vi "Dashboard Main.vi"() -> ()   [LabVIEW 2017]
uses:
  <vilib>/Utility/miscctls.llb/LVRowAndColumnTypeDef.ctl
  <vilib>/event_ctls.llb/eventvkey.ctl
  <vilib>/Rock Robotics/Network Tables/NT Read Numeric Array.vi
  <vilib>/Rock Robotics/WPI/Dashboard/WPI_DashboardLogging Global.vi
panel:
  in  "Camera Settings Right":T1={"Frame Rate"=30, "Compression"=30, "Size"=1, "DB Camera Config"=FALSE} {"Frame Rate" scale=1.0..30.0; "Compression" scale=100.0..-1.0; "Size" items=["640x480", "320x240", "160x120"]}
  in  "Camera Name Right":string(combo)="No Camera Selection"
  out "Camera Info":cluster{"Mbps LED":bool, "Mbps":dbl, "fps":dbl} {"fps" format="%#.1g"; "Mbps" format="%#.1g"}
  in  "Camera Settings":T1={"Frame Rate"=30, "Compression"=30, "Size"=1, "DB Camera Config"=FALSE} {"Frame Rate" scale=1.0..30.0; "Compression" scale=100.0..-1.0; "Size" items=["640x480", "320x240", "160x120"]}
  in  "TCP":refnum<k5>
  in  "Rec Mode":enum32{"Stop", "Record", "Playback"}(radio)
  out "Robot IP":string
  out "Image Message":string="Timeout in Camera Communications"
  in  "Dashboard Tab":T2(tab)
  in  "Select Auto":string(combo)="Select Autonomous ..."
  out "NT Connection":bool
  out "MotorChart R":cluster{"Numeric":dbl, "Numeric":dbl}(graph)
  out "MotorChart L":cluster{"Numeric":dbl, "Numeric":dbl}(graph)
  out "MotorSliders R":cluster{"MotorSlide1":dbl, "MotorSlide2":dbl} {"MotorSlide2" scale=-1.0..1.0 scale format="%#_2e"; "MotorSlide1" scale=-1.0..1.0 scale format="%#_2e"}
  out "MotorSliders L":cluster{"MotorSlide1":dbl, "MotorSlide2":dbl} {"MotorSlide2" scale=-1.0..1.0 scale format="%#_2e"; "MotorSlide1" scale=-1.0..1.0 scale format="%#_2e"}
  out "JS1 Z":dbl(slide) scale=-1.0..1.0 scale format="%#_2e"
  out "JS1 Graph":cluster{"X":dbl, "Y":dbl}[](graph)
  out "JS1 Buttons":T3
  out "JS2 Z":dbl(slide) scale=-1.0..1.0 scale format="%#_2e"
  out "JS2 Graph":cluster{"X":dbl, "Y":dbl}[](graph)
  out "JS2 Buttons":T3
  out "Mode":T4(ring)=enum."Auto Disabled"
  out "Gear State":string="Waiting...."
  out "Camera Image Right":T5(plugin-control)
  in  "DB/String 9":string
  in  "DB/String 8":string
  in  "DB/String 7":string
  in  "DB/String 6":string
  in  "DB/String 5":string
  in  "DB/String 4":string
  in  "DB/String 3":string
  in  "DB/String 2":string
  in  "DB/String 1":string
  in  "DB/String 0":string
  in  "DB/Slider 0":dbl(slide) scale=0.0..5.0
  in  "DB/Slider 1":dbl(slide) scale=0.0..5.0
  in  "DB/Slider 2":dbl(slide) scale=0.0..5.0
  in  "DB/Slider 3":dbl(slide) scale=0.0..5.0
  out "DB/LED 3":bool
  out "DB/LED 2":bool
  out "DB/LED 1":bool
  out "DB/LED 0":bool
  in  "DB/Button 3":bool
  in  "DB/Button 2":bool
  in  "DB/Button 1":bool
  in  "DB/Button 0":bool caption="New Name"
  in  "Test Slider":dbl(slide) scale=0.0..100.0 scale format="%#_3g"
  in  "On/Off":bool caption="Solenoid"
  in  "Test Name":u16(ring) items=["Select the test to run..."]
  in  "Test Tree":string(tree)
  in  "Motor":cluster{"Value":dbl, "Enable":bool} {"Value" scale=-1.0..1.0 scale format="%#_3g"}
  out "Progress":T6 {"Test Progress" scale=0.0..100.0}
  in  "Rev/Fwd":cluster{"Forward":bool, "Reverse":bool}
  in  "Test Ring":u16(ring) items=["Monochrome", "Color"]
  out "Cmd Status":string
  in  "Execute Command":bool
  in  "Command Params":string[][](table)
  in  "Command Selection":i32(listbox)
  in  "CheckList":i32(listbox)
  out "Tree":string(tree)
  out "Camera Image":T5(plugin-control)
  out "Background":bool
  in  "Camera Name":string(combo)="No Camera Selection"
  # "HW"
  # "HW"
  # "Joysticks"
  # "Drive Motors"
  # "Front"
  # "Right"
  # "Left"
  # "Back"
  # "This tab is a great place for autonomous settings and robot-specific values.\nPlace controls and indicators inside this tab and match name to\nDashboard Variables on robot. You can also delete this comment."
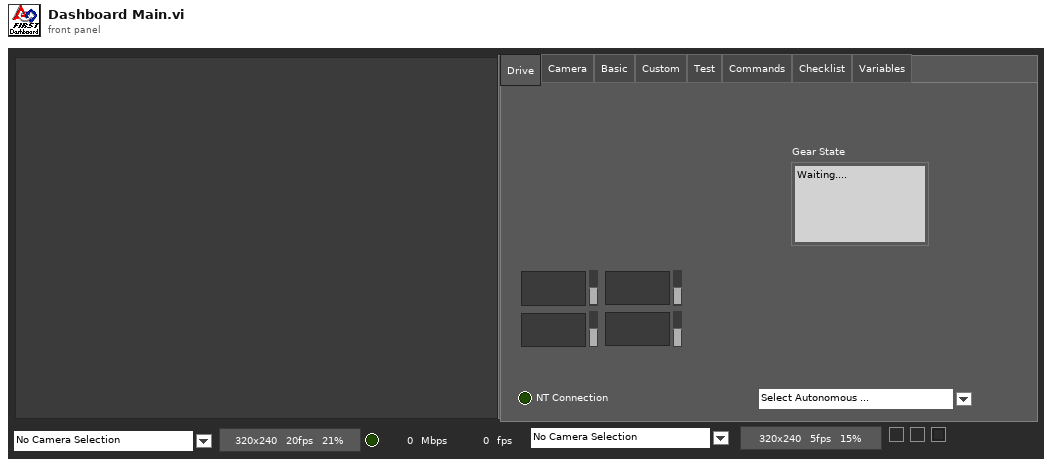
[diagram p1: front panel]
types:
  T1 = cluster{"Frame Rate":i32, "Compression":i32, "Size":u16, "DB Camera Config":bool}
  T2 = enum32{"Drive", "Camera", "Basic", "Custom", "Test", "Commands", "Checklist", "Variables"}
  T3 = cluster{bool, bool, bool, bool, bool, bool, bool, bool, bool, bool, bool, bool}
  T4 = enum8{"Tele-Op Disabled", "Tele-Op Enabled", "Auto Disabled", "Auto Enabled", "Test Disabled", "Test Enabled", "Disconnected", "No Code", "E-Stop"}
  T5 = typedef "IMAQ Image.ctl" = refnum<image>
  T6 = cluster{"Test Progress":u8, "Test Progress Text":string}
  T7 = cluster{"Save Path":path, "Interval (s)":dbl, "Keep":i32}
  T8 = typedef "Image Type" = u32
  T9 = cluster{"IDs":cluster{"RPC field ID":u16, "Unique ID":u16}, "String":string}
  T10 = cluster{"Error Strings":string, "Disable Counts":cluster{u16, u16}, "Rail Faults":cluster{u16, u16, u16}, "Robot IP":string, "DB Mode":u8, "Event Info":cluster{"Name":string, "Type":u8, "Number":u16, "Replay":u8}}
  T11 = cluster{"Storage":cluster{"Disk Free":u64, "RAM Block":u32, "RAM free":u32}, "CPU Utilization":cluster{"CPU % ISR":sgl, "CPU % Time Crit":sgl, "CPU % Timed Str":sgl, "CPU % High":sgl, "CPU % Above":sgl, "CPU % Normal":sgl, "CPU % Low":sgl}, "CAN":cluster{"% Bus Utilization":sgl, "Bus Off Cnt":u32, "TX_FIFO Full Cnt":u32, "Receive Error Cnt":u8, "Transmit Error Cnt":u8}, "HID":cluster{"HID Outputs":u32, "Rumble Low":u16, "Rumble High":u16}[]}
  T12 = cluster{"Status bits":cluster{"Test Mode":bool, "Autonomous":bool, "Enabled":bool, "Code Start":bool, "Brownout":bool, "Reserved 2":bool, "Reserved 3":bool, "E-Stop":bool}, "Code Trace":cluster{"Disabled":bool, "TeleOp":bool, "Auto":bool, "Test":bool}, "Controller Type":enum16{"unknown", "cRIO", "roboRio"}, "Code?":enum16{"unknown", "noCode", "code"}, "Battery V":dbl}
  T13 = cluster{"Control Bits":cluster{"TestMode":bool, "Autonomous":bool, "Enabled":bool, "FMS Present":bool, bool, bool, bool, "E-Stop":bool}, "Team Station ":u8, "Countdown":sgl, "Joystick Values":cluster{"Axes":dbl[], "Buttons":bool[], "POVs":i16[]}[]}
  T14 = cluster{"Axes":dbl[], "Buttons":bool[], "POVs":i16[]}[]
  T15 = cluster{"Axes":dbl[], "Buttons":bool[], "POVs":i16[]}
  T16 = cluster{"Buttons[0]":bool, "Buttons[1]":bool, "Buttons[2]":bool, "Buttons[3]":bool, "Buttons[4]":bool, "Buttons[5]":bool, "Buttons[6]":bool, "Buttons[7]":bool, "Buttons[8]":bool, "Buttons[9]":bool, "Buttons[10]":bool, "Buttons[11]":bool}
  T17 = cluster{"Camera Image":refnum<vi>, "Dashboard Tab":refnum<vi>, "Background":refnum<vi>, "Rec Mode":refnum<vi>, "Test Slider":refnum<vi>, "On/Off ":refnum<vi>, "Test Ring":refnum<vi>, "Rev/Fwd":refnum<vi>, "Test Name":refnum<vi>, "Motor":refnum<vi>, "Progress":refnum<vi>, "CheckList":refnum<vi>, "Tree":refnum<vi>, "Test Tree":refnum<vi>, "Command Params":refnum<vi>, "Command Selection":refnum<vi>, "Execute Command":refnum<vi>, "Cmd Status":refnum<vi>, "Camera Settings":refnum<vi>, "Camera Name":refnum<vi>, "Camera Info":refnum<vi>, "Camera Settings Right":refnum<vi>, "Camera Name Right":refnum<vi>, "Camera Image Right":refnum<vi>}
  T18 = cluster{"Camera Name":string, string, "Saved DB Images Info":cluster{"Save Path":path, "Interval (s)":dbl, "Keep":i32}}
  T19 = cluster{"Camera Name Right":string, string, "Saved DB Images Info":cluster{"Save Path":path, "Interval (s)":dbl, "Keep":i32}}
  T20 = cluster{"Operation":enum16{"Update", "Clear"}, "Color Box":u32}[]
  T21 = typedef "eventvkey.ctl" = enum16{"ASCII", "Enter", "Return", "Shift", "Ctrl", "Alt", "Cmd", "Opt", "Caps", "NumLock", "Clear", "Break", "Up", "Down", "Left", "Right", "Insert", "Delete", "Home", "End", "PageUp", "PageDown", "Escape", "Help", "Pause", "ScrollLock", "F1", "F2", "F3", "F4", "F5", "F6", "F7", "F8", "F9", "F10", "F11", "F12", "F13", "F14", "F15", "F16", "F17", "F18", "F19", "F20", "F21", "F22", "F23", "F24", "Play", "VolumeUp", "VolumeDown", "Mute", "Two Byte Char"}
  T22 = cluster{"Image Size":bool, "Image Type":bool, "Pixel Value":bool, "ROI Information":bool, "Zoom Factor":bool}
  T23 = cluster{"Operation":enum16{"Update", "Clear"}, "Color Box":u32}
  T24 = typedef "LVRowAndColumnTypeDef.ctl" = cluster{"Row":i32, "Column":i32}
  T25 = cluster{"Shift":bool, "Ctrl":bool, "Alt":bool, "Cmd":bool, "Opt":bool}
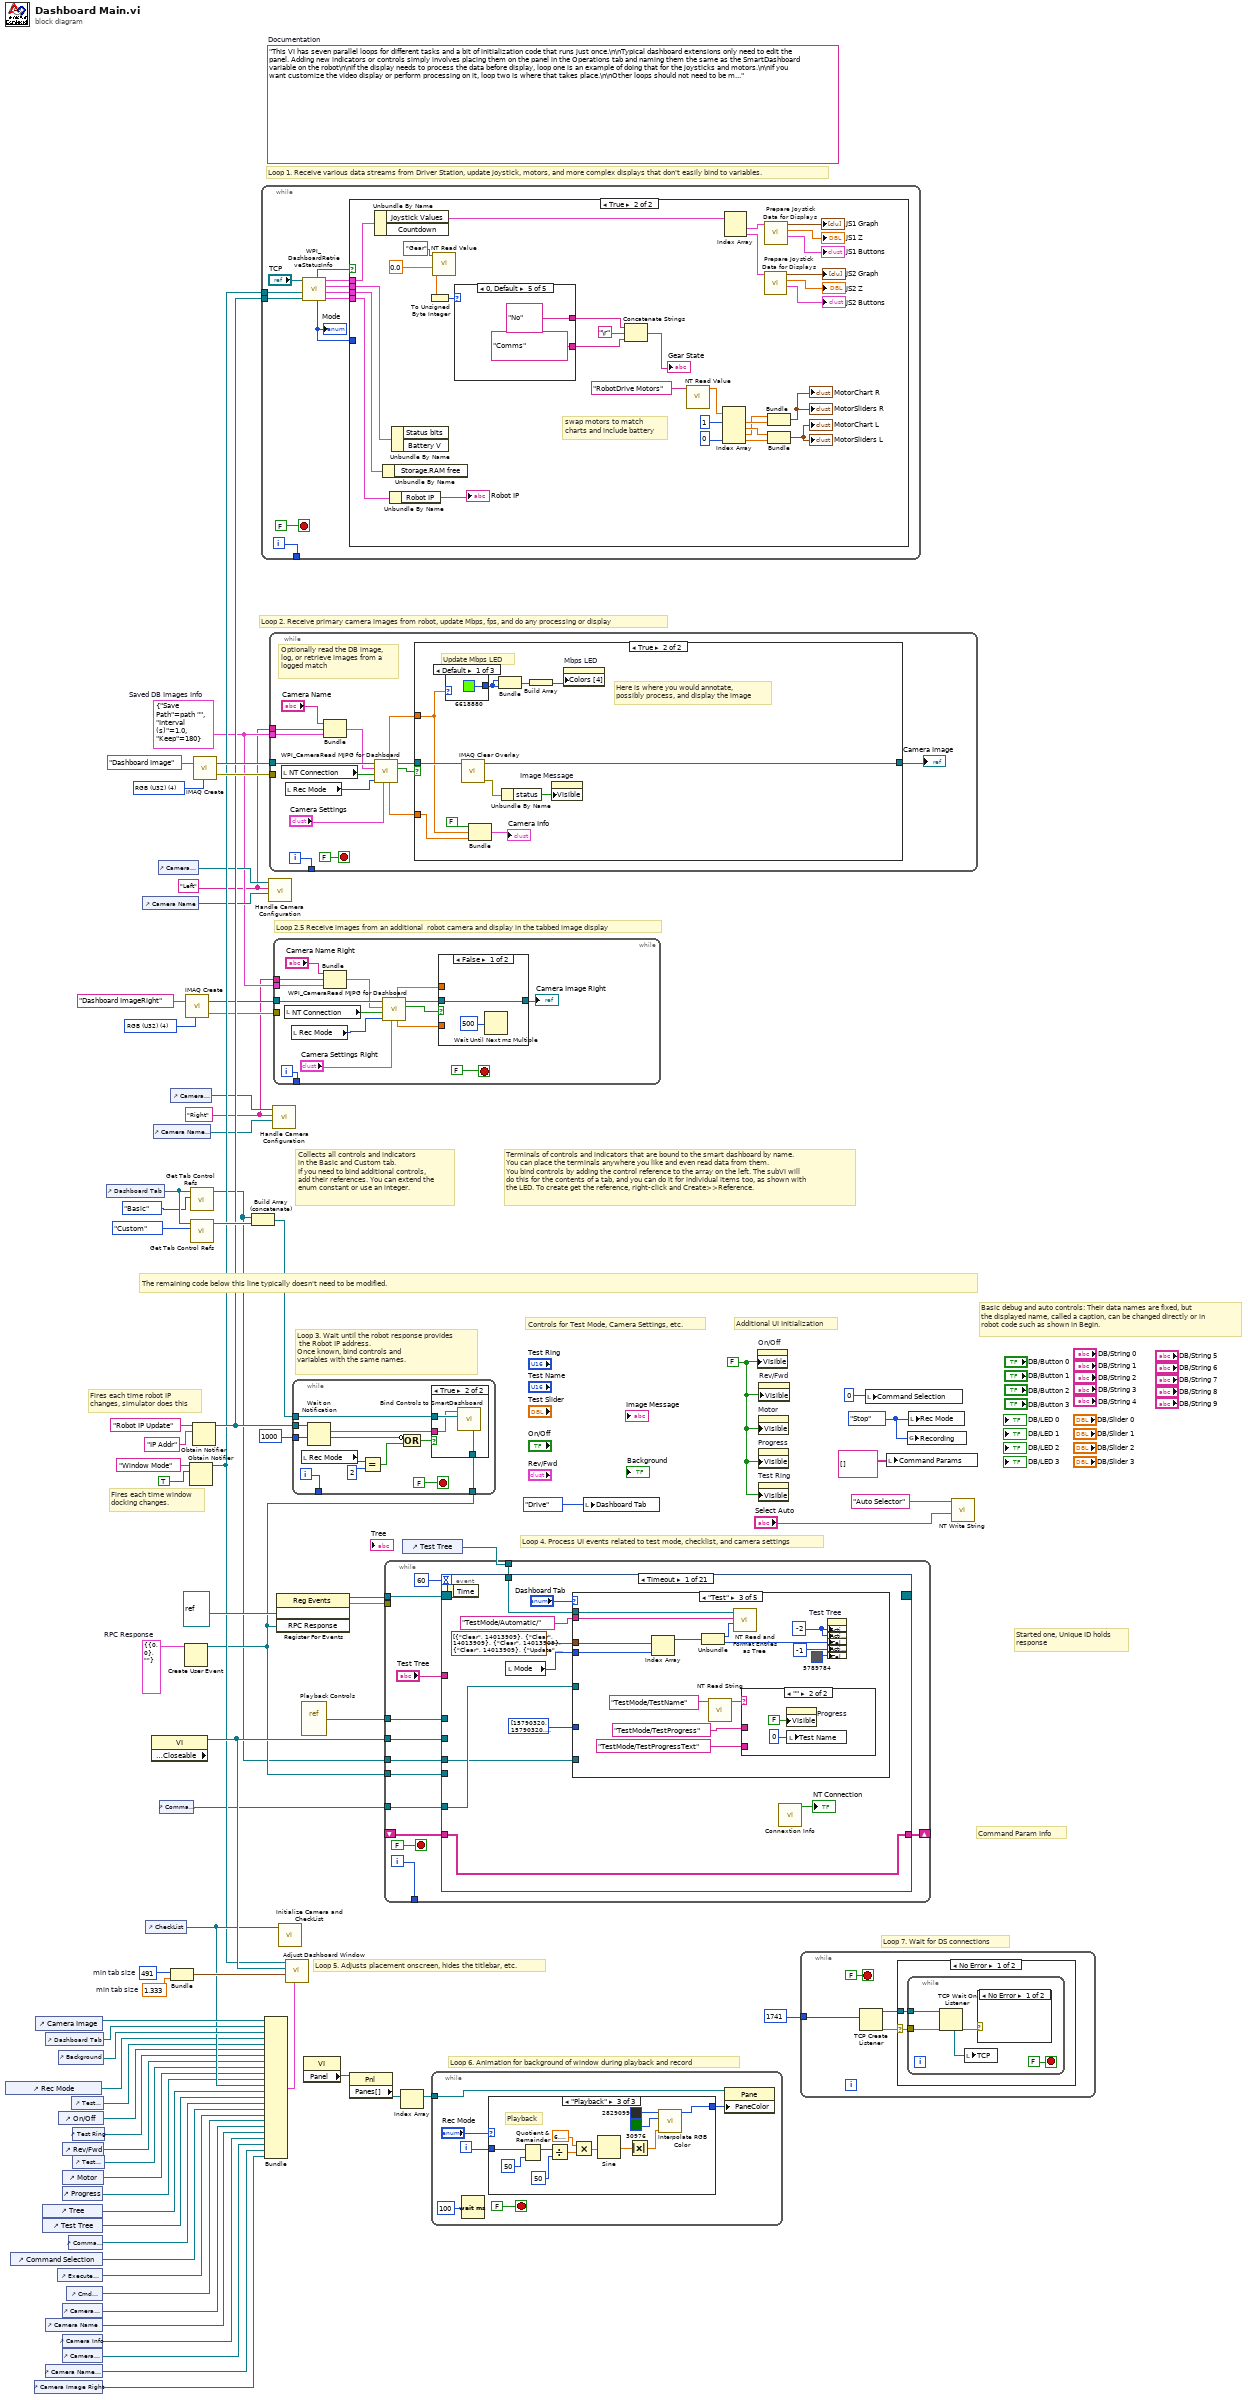
[diagram p0: block diagram]
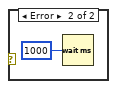
[diagram p3: hidden frame]
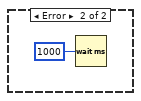
[diagram p4: hidden frame]
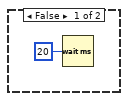
[diagram p5: hidden frame]
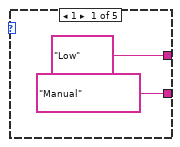
[diagram p6: hidden frame]
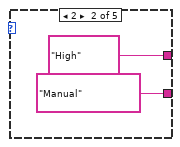
[diagram p7: hidden frame]
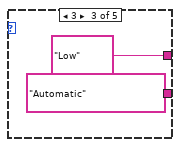
[diagram p8: hidden frame]
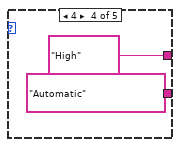
[diagram p9: hidden frame]
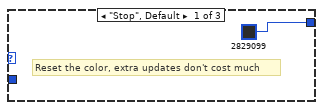
[diagram p10: hidden frame]
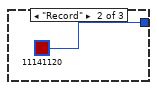
[diagram p11: hidden frame]
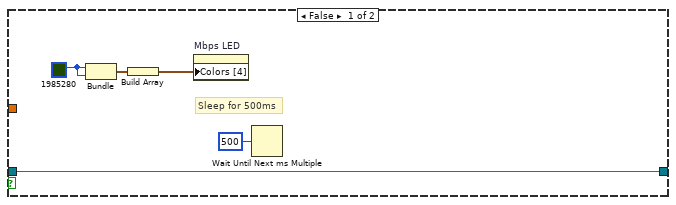
[diagram p13: hidden frame]
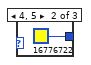
[diagram p14: hidden frame]
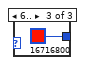
[diagram p15: hidden frame]
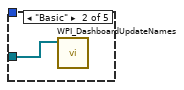
[diagram p17: hidden frame]
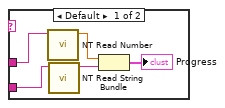
[diagram p18: hidden frame]
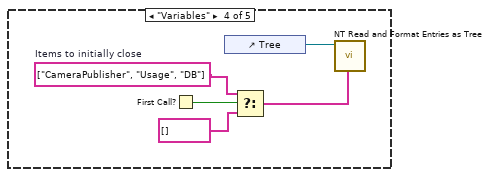
[diagram p19: hidden frame]
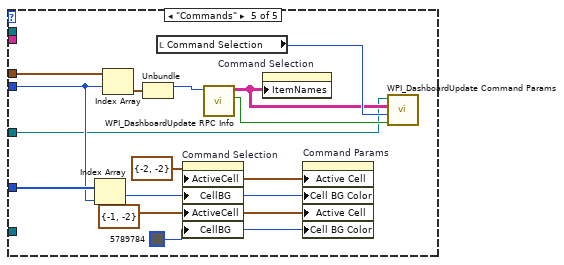
[diagram p20: hidden frame]
diagram:
  w3 = T7 {"Save Path"=path "", "Interval (s)"=1.0, "Keep"=180}  # Saved DB Images Info
  w2 = "Right"
  w1 = "Left"
  w13 = T8 4 items=["Grayscale (U8)", "Grayscale (I16)", "Grayscale (SGL)", "Complex (CSG)", "RGB (U32)", "HSL (U32)", "RGB (U64)"] ("Image Type")
  w29 = T9 {"IDs"={"RPC field ID"=0, "Unique ID"=0}, "String"=""}  # RPC Response
  w52 = 491  # min tab size
  w51 = 1.333  # min tab size
  w59 = enum32{"Stop", "Record", "Playback"}."Stop" ("Rec Mode")
  w36 = FALSE ("Visible")
  (unwired) "This VI has seven parallel loops for different tasks and a bit of initialization code that runs just once.\n\nTypical dashboard extensions only need to edit the panel. Adding new indicators or controls simply involves placing them on the panel in the Operations tab and naming them the same as the SmartDashboard variable on the robot\n\nIf the display needs to process the data before display, loop one is an example of doing that for the joysticks and motors.\n\nIf you want customize the video display or perform processing on it, loop two is where that takes place.\n\nOther loops should not need to be modified. They are pretty standard, and document the task they perform."  # Documentation
  w76 = T8 4 items=["Grayscale (U8)", "Grayscale (I16)", "Grayscale (SGL)", "Complex (CSG)", "RGB (U32)", "HSL (U32)", "RGB (U64)"] ("Image Type")
  # "Loop 2.5 Receive images from an additional  robot camera and display in the tabbed image display"
  # "Command Param Info"
  # "Started one, Unique ID holds\nresponse"
  # "Loop 7. Wait for DS connections"
  # "Basic debug and auto controls: Their data names are fixed, but\nthe displayed name, called a caption, can be changed directly or in\nrobot code such as shown in Begin."
  # "Controls for Test Mode, Camera Settings, etc."
  # "Additional UI Initialization"
  # "Loop 6. Animation for background of window during playback and record"
  # "Fires each time robot IP\nchanges, simulator does this"
  # "Fires each time window\ndocking changes."
  # "Collects all controls and indicators\nin the Basic and Custom tab.\nIf you need to bind additional controls,\nadd their references. You can extend the\nenum constant or use an integer."
  # "The remaining code below this line typically doesn't need to be modified."
  # "Loop 4. Process UI events related to test mode, checklist, and camera settings"
  # "Terminals of controls and indicators that are bound to the smart dashboard by name.\nYou can place the terminals anywhere you like and even read data from them.\nYou bind controls by adding the control reference to the array on the left. The subVI will\ndo this for the contents of a tab, and you can do it for individual items too, as shown with\nthe LED. To create get the reference, right-click and Create>>Reference."
  # "Loop 3. Wait until the robot response provides\n the Robot IP address.\nOnce known, bind controls and\nvariables with the same names."
  # "Loop 5. Adjusts placement onscreen, hides the titlebar, etc."
  # "Loop 1. Receive various data streams from Driver Station, update joystick, motors, and more complex displays that don't easily bind to variables."
  # "Loop 2. Receive primary camera images from robot, update Mbps, fps, and do any processing or display"
  n1 = control-ref of="Rec Mode"() -> (w42:refnum<vi>)
  n2 = control-ref of="Command Selection"() -> (w28:refnum<vi>)
  n3 = control-ref of="Camera Image Right"() -> (w6:refnum<vi>)
  n4 = control-ref of="Camera Image"() -> (w54:refnum<vi>)
  n5 = control-ref of="Tree"() -> (w46:refnum<vi>)
  n6 = control-ref of="Test Tree"() -> (w45:refnum<vi>)
  n7 = control-ref of="Dashboard Tab"() -> (w53:refnum<vi>)
  n8 = control-ref of="Camera Name"() -> (w19:refnum<vi>)
  n9 = control-ref of="Camera Name Right"() -> (w7:refnum<vi>)
  n10 = control-ref of="Execute Command"() -> (w30:refnum<vi>)
  n11 = control-ref of="Background"() -> (w49:refnum<vi>)
  n12 = control-ref of="On/Off"() -> (w40:refnum<vi>)
  n13 = control-ref of="Progress"() -> (w37:refnum<vi>)
  n14 = control-ref of="Camera Settings"() -> (w20:refnum<vi>)
  n15 = control-ref of="Camera Info"() -> (w18:refnum<vi>)
  n16 = control-ref of="Camera Settings Right"() -> (w8:refnum<vi>)
  n17 = control-ref of="Rev/Fwd"() -> (w38:refnum<vi>)
  n18 = control-ref of="Motor"() -> (w43:refnum<vi>)
  n19 = control-ref of="Cmd Status"() -> (w24:refnum<vi>)
  n20 = control-ref of="Command Params"() -> (w31:refnum<vi>)
  n21 = control-ref of="Test Slider"() -> (w41:refnum<vi>)
  n22 = control-ref of="Test Ring"() -> (w39:refnum<vi>)
  n23 = control-ref of="Test Name"() -> (w44:refnum<vi>)
  n24 = control-ref of="Dashboard Tab"() -> (w57:refnum<vi>)
  n25 = control-ref of="Camera Name"() -> (w21:refnum<vi>)
  n26 = control-ref of="CheckList"() -> (w47:refnum<vi>)
  n27 = property class="VI" props=["Front Panel.Closeable"]() -> (reference out=w58:refnum<vi>)  [unwired: 2 in, 2 out]
  n28 = control-ref of="Camera Name Right"() -> (w9:refnum<vi>)
  n29 = control-ref of="Camera Settings"() -> (w22:refnum<vi>)
  n30 = control-ref of="Command Params"() -> (w23:refnum<vi>)
  n31 = control-ref of="Camera Settings Right"() -> (w10:refnum<vi>)
  n32 = Bundle("min tab size"=w52, "min tab size"=w51) -> (w50:cluster{"min tab size":i32, "min tab size":dbl})  [unwired: 1 in]
  n33 = Create User Event(user event datatype=w29) -> (user event=w25:refnum<user-event>)  [unwired: 1 in, 1 out]
  n34 = call "IMAQ Create"("Image Name"="Dashboard ImageRight", "Image Type"=w13) -> ("New Image"=w12:T5, "error out"=w11:errorcluster)  [unwired: 2 in, 1 out]
  n35 = Obtain Notifier(name (unnamed)="Window Mode", notification data type=TRUE) -> (notifier out=w34:refnum<notifier>)  [unwired: 2 in, 2 out]
  n36 = call <vilib>:"Get Tab Control Refs.vi"("Page Index"=T2."Basic" ("Dashboard Tab"), "TabControl in"=w57) -> ("ControlsOnPage"=w17:refnum<vi>[])  [unwired: 9 in]
  n37 = call <vilib>:"Get Tab Control Refs.vi"("Page Index"=T2."Custom" ("Dashboard Tab"), "TabControl in"=w57) -> ("ControlsOnPage"=w56:refnum<vi>[])  [unwired: 9 in]
  n38 = Obtain Notifier(name (unnamed)="Robot IP Update", notification data type="IP Addr" ("name (unnamed)")) -> (notifier out=w35:refnum<notifier>)  [unwired: 2 in, 2 out]
  n39 = call "IMAQ Create"("Image Name"="Dashboard Image", "Image Type"=w76) -> ("New Image"=w74:T5, "error out"=w73:errorcluster)  [unwired: 2 in, 1 out]
  n40 = Build Array (concatenate)(w17, w56) -> (w55:refnum<vi>[])
  n41 = while {
    tunnel: [w86] -> _
    tunnel: w35 -> [w80]
    tunnel: w34 -> [w77]
    i -> [w86]
    stop <- FALSE stop-if-true
    n42 = call <vilib>:"WPI_DashboardRetrieveStatusInfo.vi"("Binding Refnum"=w80, "Window Mode Notifier"=w77, "TCP Cnx"="TCP") -> ("Power and Errors"=w81:T10, "Robot Metrics"=w84:T11, "Status Info"=w85:T12, "Control Info"=w82:T13, "Robot Mode"=w79:T4, "Process?"=w83:bool)  [unwired: 3 in]
    "Mode" <- w79
    n43 = case shown="True" w83 {
      tunnel: w85 -> [_ w120]
      tunnel: w84 -> [_ w119]
      tunnel: w82 -> [_ w118]
      tunnel: w81 -> [_ w117]
      tunnel: w79 -> [_ _]
      frame False {
        n44 = Wait (ms)(milliseconds to wait=u32 20) -> ()  [unwired: 1 out]
      }
      frame True {
        # "swap motors to match\ncharts and include battery"
        n45 = Unbundle By Name(w118) -> ("Joystick Values"=w108:T14)  [unwired: 1 out]
        n46 = Unbundle By Name(w119) -> ()  [unwired: 1 out]
        n47 = Unbundle By Name(w117) -> ("Robot IP"=→"Robot IP":string)
        n48 = Unbundle By Name(w120) -> ()  [unwired: 2 out]
        n49 = call-poly <vilib>:"NT Read Value.vi"("Default Value"=0.0, "Name"="Gear") -> ("Numeric"=w90:dbl)  [unwired: 8 in, 1 out]
        n50 = To Unsigned Byte Integer(number=w90) -> (unsigned 8bit integer=w89:u8)
        n51 = case shown="0, Default" w89 {
          tunnel: ["Low" "High" "Low" "High" "No"] -> w93
          tunnel: ["Manual" "Manual" "Automatic" "Automatic" "Comms"] -> w95
          frame 1 {
          }
          frame 2 {
          }
          frame 3 {
          }
          frame 4 {
          }
          frame 0, Default {
          }
        }
        n52 = Concatenate Strings(w93, "\r", w95) -> (→"Gear State":string)
        n53 = call-poly <vilib>:"NT Read Value.vi"("Name"="RobotDrive Motors") -> ("Numeric Array"=w98:dbl[])  [unwired: 9 in, 1 out]
        n54 = Index Array(array=w98, index #1=1, index #4=0) -> (element #1=w112:dbl, element #2=w113:dbl, element #3=w111:dbl, element #4=w116:dbl)  [unwired: 2 in]
        n55 = Index Array(array=w108) -> (element #1=w107:T15, element #2=w103:T15)  [unwired: 2 in]
        n56 = call "Prepare Joystick Data for Displays.vi"("Joystick Values"=w103) -> ("Buttons"=→"JS2 Buttons":T16, "Z Axis"=→"JS2 Z":dbl, "Cartesian Data"=→"JS2 Graph":cluster{"X axis":dbl, "X axis":dbl}[])  [unwired: 8 in]
        n57 = call "Prepare Joystick Data for Displays.vi"("Joystick Values"=w107) -> ("Buttons"=→"JS1 Buttons":T16, "Z Axis"=→"JS1 Z":dbl, "Cartesian Data"=→"JS1 Graph":cluster{"X axis":dbl, "X axis":dbl}[])  [unwired: 8 in]
        n58 = Bundle("Numeric"=w111, "Numeric"=w112) -> (→"MotorChart R" →"MotorSliders R":cluster{"Numeric":dbl, "Numeric":dbl})  [unwired: 1 in]
        n59 = Bundle("Numeric"=w113, "Numeric"=w116) -> (→"MotorChart L" →"MotorSliders L":cluster{"Numeric":dbl, "Numeric":dbl})  [unwired: 1 in]
      }
    }
  }
  n60 = Bundle("Camera Image"=w54, "Dashboard Tab"=w53, "Background"=w49, "Rec Mode"=w42, "Test Slider"=w41, "On/Off"=w40, "Test Ring"=w39, "Rev/Fwd"=w38, "Test Name"=w44, "Motor"=w43, "Progress"=w37, "CheckList"=w47, "Tree"=w46, "Test Tree"=w45, "Command Params"=w31, "Command Selection"=w28, "Execute Command"=w30, "Cmd Status"=w24, "Camera Settings"=w20, "Camera Name"=w19, "Camera Info"=w18, "Camera Settings Right"=w8, "Camera Name Right"=w7, "Camera Image Right"=w6) -> (w48:T17)  [unwired: 1 in]
  n61 = call "Handle Camera Configuration.vi"("CameraNameRef"=w21, "Display Name"=w1, "ClusterRef"=w22) -> ()  [unwired: 9 in]
  n62 = while {
    tunnel: w74 -> [w143]
    tunnel: w73 -> [_]
    tunnel: [w144] -> _
    tunnel: w3 -> [w134]
    tunnel: w1 -> [w131]
    i -> [w144]
    stop <- FALSE stop-if-true
    # "Optionally read the DB image,\nlog, or retrieve images from a\nlogged match"
    n63 = local read "NT Connection"() -> (w135:bool)
    n64 = local read "Rec Mode"() -> (w139:enum32{"Stop", "Record", "Playback"})
    n65 = Bundle("Camera Name"="Camera Name", w131, "Saved DB Images Info"=w134) -> (w133:T18)  [unwired: 1 in]
    n66 = call <vilib>:"WPI_CameraRead MJPG for Dashboard.vi"("Camera Settings"="Camera Settings", "Rec Mode"=w139, "NT Connection"=w135, "Capture Info"=w133, "Refnum in"=w143) -> ("Active"=w141:bool, "Refnum out"=w142:T5, "FPS"=w140:dbl, "Bandwidth (Mbps)"=w138:dbl)  [unwired: 3 in]
    n67 = case shown="True" w141 {
      tunnel: w142 -> [w146 w157]
      tunnel: w138 -> [_ w154]
      tunnel: w140 -> [_ w155]
      tunnel: [w146 w151] -> w136
      frame False {
        w148 = u32 1985280 ("Color Box")
        # "Sleep for 500ms"
        n68 = Bundle("Color Box"=w148, "Color Box"=w148) -> (w149:cluster{"Color Box":u32, "Color Box":u32})  [unwired: 1 out]
        n69 = Build Array(w149) -> (w147:cluster{"Color Box":u32, "Color Box":u32}[])
        n70 = property on="Mbps LED" class="Bool (strict)"("Colors [4]"=w147) -> ()  [unwired: 2 in, 2 out]
        n71 = Wait Until Next ms Multiple(millisecond multiple=u32 500) -> ()  [unwired: 1 out]
      }
      frame True {
        # "Here is where you would annotate,\npossibly process, and display the image"
        # "Update Mbps LED"
        n72 = case shown="Default" w154 {
          tunnel: [u32 6618880 ("Color Box") u32 16776722 ("Color Box") u32 16716800 ("Color Box")] -> w158
          frame Default {
          }
          frame 4, 5 {
          }
          frame 6.. {
          }
        }
        n73 = call "IMAQ Clear Overlay"("Image"=w157) -> ("error out"=w160:errorcluster, "Image Out"=w151:T5)  [unwired: 2 in, 7 out]
        n74 = Bundle(FALSE, "Bandwidth (Mbps)"=w154, "FPS"=w155) -> (→"Camera Info":cluster{bool, "Bandwidth (Mbps)":dbl, "FPS":dbl})  [unwired: 1 in]
        n75 = Bundle("Color Box"=w158, "Color Box"=w158) -> (w159:cluster{"Color Box":u32, "Color Box":u32})  [unwired: 1 out]
        n76 = Unbundle By Name(w160) -> ("status"=w161:bool)
        n77 = Build Array(w159) -> (w156:cluster{"Color Box":u32, "Color Box":u32}[])
        n78 = property on="Image Message" class="Str"("Visible"=w161) -> ()  [unwired: 2 in, 2 out]
        n79 = property on="Mbps LED" class="Bool (strict)"("Colors [4]"=w156) -> ()  [unwired: 2 in, 2 out]
      }
    }
    "Camera Image" <- w136
  }
  n80 = call "Handle Camera Configuration.vi"("CameraNameRef"=w9, "Display Name"=w2, "ClusterRef"=w10) -> ()  [unwired: 9 in]
  n81 = while {
    tunnel: w12 -> [w179]
    tunnel: w11 -> [_]
    tunnel: [w174] -> _
    tunnel: w3 -> [w168]
    tunnel: w2 -> [w165]
    i -> [w174]
    stop <- FALSE stop-if-true
    n82 = local read "NT Connection"() -> (w169:bool)
    n83 = local read "Rec Mode"() -> (w178:enum32{"Stop", "Record", "Playback"})
    n84 = Bundle("Camera Name Right"="Camera Name Right", w165, "Saved DB Images Info"=w168) -> (w167:T19)  [unwired: 1 in]
    n85 = call <vilib>:"WPI_CameraRead MJPG for Dashboard.vi"("Camera Settings"="Camera Settings Right", "Rec Mode"=w178, "NT Connection"=w169, "Capture Info"=w167, "Refnum in"=w179) -> ("Active"=w173:bool, "Refnum out"=w176:T5, "FPS"=w171:dbl, "Bandwidth (Mbps)"=w172:dbl)  [unwired: 3 in]
    n86 = case shown="False" w173 {
      tunnel: w176 -> [w180 w182]
      tunnel: w172 -> [_ _]
      tunnel: w171 -> [_ _]
      tunnel: [w180 w182] -> w170
      frame False {
        n87 = Wait Until Next ms Multiple(millisecond multiple=u32 500) -> ()  [unwired: 1 out]
      }
      frame True {
      }
    }
    "Camera Image Right" <- w170
  }
  n88 = register-events(refnum<vi> refnum, w25) -> (reference out=w63:refnum<event-registration>, error out=w62:errorcluster)  [unwired: 2 in]
  n89 = call "Initialize Camera and CheckList.vi"("ListBox in"=w47) -> ()  [unwired: 11 in]
  n90 = call "Adjust Dashboard Window.vi"("Sizing Refnums"=w48, "Size Constraints"=w50, "VI"=w58, "WIn Mode"=w34) -> ()  [unwired: 8 in]
  n91 = while {
    tunnel: w55 -> [w194]
    tunnel: w35 -> [w192]
    tunnel: [w190] -> _
    tunnel: u32 1000 ("milliseconds to wait") -> [w189]
    tunnel: w25 -> [w183]
    i -> [w190]
    stop <- FALSE stop-if-true
    n92 = local read "Rec Mode"() -> (w185:enum32{"Stop", "Record", "Playback"})
    n93 = Wait on Notification(notifier=w192, timeout in ms (-1)=w189) -> (notification=w191:string, timed out?=w187:bool)  [unwired: 2 in, 2 out]
    n94 = Equal?(x=w185, y=u16 2 ("Rec Mode")) -> (x = y?=w186:bool)
    n95 = Compound Arithmetic op=OR(invert w187, w186) -> (w188:bool)
    n96 = case shown="True" w188 {
      tunnel: w194 -> [_ w197]
      tunnel: w191 -> [_ w196]
      tunnel: w183 -> [_ w195]
      frame False {
      }
      frame True {
        n97 = call <vilib>:"Bind Controls to SmartDashboard.vi"("RPC ref"=w195, "Bound Control Refs"=w197, "Server IP Address"=w196) -> ()  [unwired: 9 in]
      }
    }
  }
  n98 = vi-ref "Playback Controls.vi"() -> (w64:refnum<vi>)
  n99 = property class="VI"() -> ("Panel"=w66:refnum<vi>)  [unwired: 2 in, 2 out]
  n100 = property class="Pnl"(reference=w66) -> ("Panes[]"=w67:refnum<vi>[])  [unwired: 1 in, 2 out]
  n101 = Index Array(array=w67) -> (element=w65:refnum<vi>)  [unwired: 1 in]
  n102 = control-ref of="Test Tree"() -> (w68:refnum<vi>)
  n103 = while {
    tunnel: [w207] -> _
    tunnel: w68 -> [w206]
    tunnel: w64 -> [w205]
    tunnel: w63 -> [w204]
    tunnel: w62 -> [_]
    tunnel: w58 -> [w203]
    tunnel: w25 -> [w202]
    tunnel: w23 -> [w201]
    shift-right: [w200] -> _
    shift-left: _ -> [w199]
    tunnel: w17 -> [w198]
    i -> [w207]
    stop <- FALSE stop-if-true
    n104 = event shown="[0] Timeout" {
      selector: w204 -> [_ _ _ _ _ _ _ _ _ _ _ _ _ _ _ _ _ _ _ _ _]
      dyn-events: [_ _ _ _ _ _ _ _ _ _ _ _ _ _ _ _ w467 _ _ _ _] -> _
      timeout: u32 60 ("milliseconds to wait") -> [_ _ _ _ _ _ _ _ _ _ _ _ _ _ _ _ _ _ _ _ _]
      tunnel: w206 -> [w219 _ _ _ _ _ _ _ _ _ _ _ _ _ _ _ _ _ _ _ _]
      tunnel: "Test Tree" -> [_ _ _ _ _ _ _ _ _ _ _ w434 w442 w444 w448 w456 _ _ _ _ _]
      tunnel: w205 -> [_ _ _ _ _ _ _ _ _ _ _ _ _ _ _ _ w469 _ w487 _ _]
      tunnel: w203 -> [_ _ _ _ _ _ _ _ _ _ _ _ _ _ _ _ w465 _ _ _ _]
      tunnel: w202 -> [_ _ _ _ _ _ _ _ _ _ _ _ _ _ _ _ w463 _ _ _ _]
      tunnel: w201 -> [w214 _ _ _ _ _ w385 _ _ _ _ _ _ _ _ _ _ _ _ _ _]
      tunnel: [w213 w262 w364 w369 w378 w382 w383 w392 w402 w409 w421 w433 w440 w443 w447 w455 w462 w482 w484 w488 w501] -> w200
      tunnel: w199 -> [w213 w262 w364 w369 w378 w382 w383 _ _ w409 w421 w433 w440 w443 w447 w455 w462 w482 w484 w488 w501]
      tunnel: w198 -> [w211 _ _ _ _ _ _ _ _ _ _ _ _ _ _ _ _ _ _ _ _]
      event Timeout {
        n105 = event-data() -> ()  [unwired: 1 in, 1 out]
        n106 = local read "Mode"() -> (w216:T4)
        n107 = case shown="\"Test\"" "Dashboard Tab" {
          tunnel: w219 -> [_ _ w235 _ _]
          tunnel: "TestMode/Automatic/" ("Name Pattern") -> [_ _ w234 _ _]
          tunnel: T20 [{"Operation"=enum."Clear", "Color Box"=14013909}, {"Operation"=enum."Clear", "Color Box"=14013909}, {"Operation"=enum."Clear", "Color Box"=14013909}, {"Operation"=enum."Clear", "Color Box"=14013909}, {"Operation"=enum."Update", "Color Box"=14013909}, {"Operation"=enum."Update", "Color Box"=16777215}, {"Operation"=enum."Clear", "Color Box"=14013909}, {"Operation"=enum."Clear", "Color Box"=14013909}, {"Operation"=enum."Clear", "Color Box"=14013909}] -> [_ _ w227 _ w255]
          tunnel: w216 -> [_ _ w226 _ w254]
          tunnel: u32[] [15790320, 15790320, 15790320, 15790320, 16777215, 16777215, 15790320, 15790320, 15790320] -> [_ _ _ _ w260]
          tunnel: w214 -> [_ _ _ _ w248]
          tunnel: w211 -> [_ w221 _ _ _]
          frame "Custom", Default {
          }
          frame "Basic" {
            n108 = call <vilib>:"WPI_DashboardUpdateNames.vi"("Controls on Tab"=w221) -> ()  [unwired: 11 in]
          }
          frame "Test" {
            w233 = -2 ("Active Item:Row Number")
            n109 = Index Array(array=w227, index=w226) -> (element=w228:T23)
            n110 = Unbundle(w228) -> ("Operation"=w229:enum16{"Update", "Clear"}, "Color Box"=w230:u32)
            n111 = call <vilib>:"NT Read String.vi"("Name"="TestMode/TestName") -> ("String"=w224:string)  [unwired: 9 in, 1 out]
            n112 = call <vilib>:"NT Read and Format Entries as Tree.vi"("Operation"=w229, "Name Pattern"=w234, "Tree Refnum"=w235) -> ()  [unwired: 7 in, 2 out]
            n113 = case shown="\"\"" w224 {
              tunnel: "TestMode/TestProgress" ("Name") -> [w237 _]
              tunnel: "TestMode/TestProgressText" ("Name") -> [w236 _]
              frame Default {
                n114 = call <vilib>:"NT Read Number.vi"("Name"=w237) -> ("Numeric"=w238:dbl)  [unwired: 9 in, 1 out]
                n115 = call <vilib>:"NT Read String.vi"("Name"=w236) -> ("String"=w239:string)  [unwired: 9 in, 1 out]
                n116 = Bundle("Numeric"=w238, "String"=w239) -> (→"Progress":cluster{"Numeric":dbl, "String":string})  [unwired: 1 in]
              }
              frame "" {
                n117 = property on="Progress" class="Clust (strict)"("Visible"=FALSE) -> ()  [unwired: 2 in, 2 out]
                n118 = local write "Test Name"(u16 0) -> ()
              }
            }
            n119 = property on="Test Tree" class="Tree (strict)"("Active Item Row Number"=w233, "ActiveColNum"=w233, "CellBG"=w230, "Active Item Row Number"=-1 ("Active Item:Row Number"), "CellBG"=u32 5789784 ("Color Box")) -> ()  [unwired: 2 in, 2 out]
          }
          frame "Variables" {
            w245 = string[] ["CameraPublisher", "Usage", "DB"]  # Items to initially close
            n120 = First Call?() -> (First Call?: T/F=w246:bool)
            n121 = control-ref of="Tree"() -> (w247:refnum<vi>)
            n122 = Select(t=w245, s=w246, f=string[] []) -> (s? t:f=w243:string[])
            n123 = call <vilib>:"NT Read and Format Entries as Tree.vi"("Tags to  Close"=w243, "Tree Refnum"=w247) -> ()  [unwired: 8 in, 2 out]
          }
          frame "Commands" {
            w256 = u32 5789784 ("Color Box")
            w257 = T24 {"Row"=-1, "Column"=-2} ("Active Cell:Active Cell")
            w259 = T24 {"Row"=-2, "Column"=-2} ("Active Cell:Active Cell")
            n124 = Index Array(array=w260, index=w254) -> (element=w258:u32)
            n125 = Index Array(array=w255, index=w254) -> (element=w253:T23)
            n126 = Unbundle(w253) -> ("Operation"=w252:enum16{"Update", "Clear"})  [unwired: 1 out]
            n127 = local read "Command Selection"() -> (w251:i32)
            n128 = property on="Command Selection" class="MCListbox (strict)"("ActiveCell"=w259, "CellBG"=w258, "ActiveCell"=w257, "CellBG"=w256) -> ()  [unwired: 2 in, 2 out]
            n129 = call <vilib>:"WPI_DashboardUpdate RPC Info.vi"("Operation"=w252) -> ("update"=w250:bool, "commands"=w249:string[][])  [unwired: 9 in]
            n130 = property on="Command Selection" class="MCListbox (strict)"("ItemNames"=w249) -> ()  [unwired: 2 in, 2 out]
            n131 = property on="Command Params" class="Tbl (strict)"("Active Cell"=w259, "Cell BG Color"=w258, "Active Cell"=w257, "Cell BG Color"=w256) -> ()  [unwired: 2 in, 2 out]
            n132 = call <vilib>:"WPI_DashboardUpdate Command Params.vi"("Update"=w250, "NewVal"=w251, "Commands"=w249, "Param Tbl"=w248) -> ()  [unwired: 7 in, 1 out]
          }
        }
        n133 = call <vilib>:"Connextion Info.vi"() -> ("Connected"=→"NT Connection":bool)  [unwired: 10 in, 1 out]
      }
      event "Test Tree": Value Change {
        # "Show appropriate\ncontrols"
        n134 = event-data() -> ("CtlRef"=w265:refnum<vi>, "NewVal"=w263:string)  [unwired: 1 in]
        n135 = call <vilib>:"WPI_UtilitiesGetTreeIOName.vi"("NewVal"=w263, "TreeControl in"=w265) -> ("I/O Name"=w266:string)  [unwired: 9 in]
        n136 = case shown="\"Camera\"" w266 {
          selector: w266 -> [_ w273 _ w295 w304 _]
          tunnel: w263 -> [_ _ w292 w294 _ w311]
          tunnel: cluster{string[]}[] [{["640x480", "320x240", "160x120"]}, {["Auto", "Fixed indoor", "Fixed outdoor 1", "Fixed outdoor 2", "Fixed fluorescent 1", "Fixed fluorescent 2", "Hold current"]}, {["Auto", "Flicker-free 50 Hz", "Flicker-free 60 Hz", "Hold current"]}, {["None", "Prioritize frame rate", "Prioritize image quality"]}, {["Monochrome", "Color"]}] -> [_ _ _ _ _ w310]
          frame Default {
            w268 = FALSE ("Visible")
            w267 = FALSE ("Visible")
            n137 = property on="Motor" class="Clust (strict)"("Visible"=w267) -> ()  [unwired: 2 in, 2 out]
            n138 = property on="Test Ring" class="Ring (strict)"("Visible"=w267) -> ()  [unwired: 2 in, 2 out]
            n139 = property on="Rev/Fwd" class="Clust (strict)"("Visible"=w268) -> ()  [unwired: 2 in, 2 out]
            n140 = property on="On/Off" class="Bool (strict)"("Visible"=w268) -> ()  [unwired: 2 in, 2 out]
            n141 = property on="Test Slider" class="Slide (strict)"("Visible"=w268) -> ()  [unwired: 2 in, 2 out]
          }
          frame "Analog Out", "Motor", "PWM" {
            w274 = FALSE ("Visible")
            n142 = case shown="\"Analog Out\"" w273 {
              tunnel: [1.0 ("Value") -1.0 ("Value") 0.0 ("Value")] -> w272
              tunnel: [255.0 ("Value") 1.0 ("Value") 5.0 ("Value")] -> w271
              tunnel: [128.0 ("Value") 0.0 ("Value") 0.0 ("Value")] -> w270
              tunnel: [64.0 ("Value") 0.5 ("Value") 1.0 ("Value")] -> w269
              frame "PWM" {
              }
              frame "Motor", Default {
              }
              frame "Analog Out" {
              }
            }
            n143 = property on="Motor" class="Clust (strict)"("Visible"=TRUE) -> ()  [unwired: 2 in, 2 out]
            n144 = property on="Value" class="Slide (strict)"("Value"=w270, "Scale.Minimum"=w272, "Scale.Maximum"=w271, "Scale.Increment"=w269) -> ()  [unwired: 2 in, 2 out]
            n145 = property on="On/Off" class="Bool (strict)"("Visible"=w274) -> ()  [unwired: 2 in, 2 out]
            n146 = property on="Test Slider" class="Slide (strict)"("Visible"=w274) -> ()  [unwired: 2 in, 2 out]
            n147 = property on="Test Ring" class="Ring (strict)"("Visible"=w274) -> ()  [unwired: 2 in, 2 out]
            n148 = property on="Rev/Fwd" class="Clust (strict)"("Visible"=w274) -> ()  [unwired: 2 in, 2 out]
          }
          frame "Servo" {
            w290 = FALSE ("Visible")
            n149 = call <vilib>:"NT Read Number.vi"("Name"=w292) -> ("Numeric"=w291:dbl)  [unwired: 9 in, 1 out]
            n150 = property on="Test Slider" class="Slide (strict)"("Visible"=TRUE, "Scale.Maximum"=170.0 ("Scale.Range:Maximum")) -> ()  [unwired: 2 in, 2 out]
            n151 = local write "Test Slider"(w291) -> ()
            n152 = property on="Motor" class="Clust (strict)"("Visible"=w290) -> ()  [unwired: 2 in, 2 out]
            n153 = property on="Rev/Fwd" class="Clust (strict)"("Visible"=w290) -> ()  [unwired: 2 in, 2 out]
            n154 = property on="On/Off" class="Bool (strict)"("Visible"=w290) -> ()  [unwired: 2 in, 2 out]
            n155 = property on="Test Ring" class="Ring (strict)"("Visible"=w290) -> ()  [unwired: 2 in, 2 out]
          }
          frame "Relay", "Solenoid" {
            w293 = FALSE ("Visible")
            n156 = property on="Motor" class="Clust (strict)"("Visible"=w293) -> ()  [unwired: 2 in, 2 out]
            n157 = property on="Test Slider" class="Slide (strict)"("Visible"=w293) -> ()  [unwired: 2 in, 2 out]
            n158 = Search and Replace String(input string=w294, search string="/Value  **", replace string="/Direction") -> (result string=w300:string)  [unwired: 5 in, 3 out]
            n159 = property on="Test Ring" class="Ring (strict)"("Visible"=w293) -> ()  [unwired: 2 in, 2 out]
            n160 = call <vilib>:"NT Read String.vi"("Name"=w300) -> ("String"=w298:string)  [unwired: 9 in, 1 out]
            n161 = Equal?(x="Both directions", y=w298) -> (x = y?=w296:bool)
            n162 = Not(x=w296) -> (.not. x?=w297:bool)
            n163 = property on="Rev/Fwd" class="Clust (strict)"("Visible"=w296) -> ()  [unwired: 2 in, 2 out]
            n164 = property on="On/Off" class="Bool (strict)"("Visible"=w297, "Caption.Text"=w295) -> ()  [unwired: 2 in, 2 out]
          }
          frame "Compressor", "Digital Out" {
            w303 = FALSE ("Visible")
            # "Get direction and finish"
            n165 = property on="Motor" class="Clust (strict)"("Visible"=w303) -> ()  [unwired: 2 in, 2 out]
            n166 = property on="Test Slider" class="Slide (strict)"("Visible"=w303) -> ()  [unwired: 2 in, 2 out]
            n167 = property on="Test Ring" class="Ring (strict)"("Visible"=w303) -> ()  [unwired: 2 in, 2 out]
            n168 = property on="On/Off" class="Bool (strict)"("Visible"=TRUE, "Caption.Text"=w304) -> ()  [unwired: 2 in, 2 out]
            n169 = property on="Rev/Fwd" class="Clust (strict)"("Visible"=FALSE) -> ()  [unwired: 2 in, 2 out]
          }
          frame "Camera" {
            n170 = call <vilib>:"Get Last Path Segment.vi"("String in"=w311) -> ("String out"=w312:string)  [unwired: 10 in]
            n171 = property on="On/Off" class="Bool (strict)"("Visible"=FALSE) -> ()  [unwired: 2 in, 2 out]
            n172 = property on="Motor" class="Clust (strict)"("Visible"=FALSE) -> ()  [unwired: 2 in, 2 out]
            n173 = property on="Rev/Fwd" class="Clust (strict)"("Visible"=FALSE) -> ()  [unwired: 2 in, 2 out]
            n174 = case shown="\"White Balance  **\"" w312 {
              tunnel: w311 -> [w318 w327 w336 w345 w354 _ w360]
              tunnel: w310 -> [w316 w324 w333 w342 w351 _ _]
              frame "Size  **" {
                n175 = Index Array(array=w316) -> (element=w315:cluster{string[]})  [unwired: 1 in]
                n176 = call <vilib>:"NT Read String.vi"("Name"=w318) -> ("String"=w317:string)  [unwired: 9 in, 1 out]
                n177 = Unbundle(w315) -> (w313:string[])
                n178 = Match First String(2:w313, 3:w317) -> (0:w314:i32)  [unwired: 1 out]
                n179 = property on="Test Ring" class="Ring (strict)"("Value"=w314, "Strings []"=w313) -> ()  [unwired: 2 in, 2 out]
                n180 = property on="Test Ring" class="Ring (strict)"("Visible"=TRUE) -> ()  [unwired: 2 in, 2 out]
                n181 = property on="Test Slider" class="Slide (strict)"("Visible"=FALSE) -> ()  [unwired: 2 in, 2 out]
              }
              frame "White Balance  **" {
                n182 = Index Array(array=w324, index=1) -> (element=w325:cluster{string[]})
                n183 = call <vilib>:"NT Read String.vi"("Name"=w327) -> ("String"=w326:string)  [unwired: 9 in, 1 out]
                n184 = Unbundle(w325) -> (w322:string[])
                n185 = Match First String(2:w322, 3:w326) -> (0:w321:i32)  [unwired: 1 out]
                n186 = property on="Test Ring" class="Ring (strict)"("Value"=w321, "Strings []"=w322) -> ()  [unwired: 2 in, 2 out]
                n187 = property on="Test Ring" class="Ring (strict)"("Visible"=TRUE) -> ()  [unwired: 2 in, 2 out]
                n188 = property on="Test Slider" class="Slide (strict)"("Visible"=FALSE) -> ()  [unwired: 2 in, 2 out]
              }
              frame "Exposure  **" {
                n189 = Index Array(array=w333, index=2) -> (element=w334:cluster{string[]})
                n190 = call <vilib>:"NT Read String.vi"("Name"=w336) -> ("String"=w335:string)  [unwired: 9 in, 1 out]
                n191 = Unbundle(w334) -> (w330:string[])
                n192 = Match First String(2:w330, 3:w335) -> (0:w331:i32)  [unwired: 1 out]
                n193 = property on="Test Ring" class="Ring (strict)"("Value"=w331, "Strings []"=w330) -> ()  [unwired: 2 in, 2 out]
                n194 = property on="Test Ring" class="Ring (strict)"("Visible"=TRUE) -> ()  [unwired: 2 in, 2 out]
                n195 = property on="Test Slider" class="Slide (strict)"("Visible"=FALSE) -> ()  [unwired: 2 in, 2 out]
              }
              frame "Exposure Priority  **" {
                n196 = Index Array(array=w342, index=3) -> (element=w343:cluster{string[]})
                n197 = call <vilib>:"NT Read String.vi"("Name"=w345) -> ("String"=w344:string)  [unwired: 9 in, 1 out]
                n198 = Unbundle(w343) -> (w339:string[])
                n199 = Match First String(2:w339, 3:w344) -> (0:w340:i32)  [unwired: 1 out]
                n200 = property on="Test Ring" class="Ring (strict)"("Value"=w340, "Strings []"=w339) -> ()  [unwired: 2 in, 2 out]
                n201 = property on="Test Ring" class="Ring (strict)"("Visible"=TRUE) -> ()  [unwired: 2 in, 2 out]
                n202 = property on="Test Slider" class="Slide (strict)"("Visible"=FALSE) -> ()  [unwired: 2 in, 2 out]
              }
              frame "Color Enable  **" {
                n203 = Index Array(array=w351, index=4) -> (element=w352:cluster{string[]})
                n204 = call <vilib>:"NT Read String.vi"("Name"=w354) -> ("String"=w353:string)  [unwired: 9 in, 1 out]
                n205 = Unbundle(w352) -> (w348:string[])
                n206 = Match First String(2:w348, 3:w353) -> (0:w349:i32)  [unwired: 1 out]
                n207 = property on="Test Ring" class="Ring (strict)"("Value"=w349, "Strings []"=w348) -> ()  [unwired: 2 in, 2 out]
                n208 = property on="Test Ring" class="Ring (strict)"("Visible"=TRUE) -> ()  [unwired: 2 in, 2 out]
                n209 = property on="Test Slider" class="Slide (strict)"("Visible"=FALSE) -> ()  [unwired: 2 in, 2 out]
              }
              frame Default {
                n210 = property on="Test Ring" class="Ring (strict)"("Visible"=FALSE) -> ()  [unwired: 2 in, 2 out]
                n211 = property on="Test Slider" class="Slide (strict)"("Visible"=FALSE) -> ()  [unwired: 2 in, 2 out]
              }
              frame "Brightness  **", "Color Level  **", "Compression  **", "FPS  **", "Sharpness  **" {
                n212 = call <vilib>:"NT Read Number.vi"("Name"=w360) -> ("Numeric"=w359:dbl)  [unwired: 9 in, 1 out]
                n213 = local write "Test Slider"(w359) -> ()
                n214 = property on="Test Slider" class="Slide (strict)"("Visible"=TRUE, "Scale.Maximum"=100.0 ("Scale.Range:Maximum")) -> ()  [unwired: 2 in, 2 out]
                n215 = property on="Test Ring" class="Ring (strict)"("Visible"=FALSE) -> ()  [unwired: 2 in, 2 out]
              }
            }
          }
        }
        n216 = property on="Progress" class="Clust (strict)"("Visible"=FALSE) -> ()  [unwired: 2 in, 2 out]
      }
      event "Test Name": Mouse Enter {
        # "Populate the ring with the list of tests"
        n217 = event-data() -> ()  [unwired: 1 in, 1 out]
        n218 = call <vilib>:"NT Read String Array.vi"("Name"="TestMode/TestList") -> ("String Array"=w368:string[])  [unwired: 9 in, 1 out]
        n219 = Build Array (concatenate)("Select the test to run...", w368) -> (w367:string[])
        n220 = property on="Test Name" class="Ring (strict)"("Strings []"=w367) -> ()  [unwired: 2 in, 2 out]
      }
      event "Test Name": Value Change {
        w370 = FALSE ("Visible")
        # "Tell the robot the test name to run"
        n221 = event-data() -> ("NewVal"=w374:u16)  [unwired: 1 in]
        n222 = property on="Test Name" class="Ring (strict)"() -> ("Strings []"=w375:string[])  [unwired: 2 in, 2 out]
        n223 = local write "Progress"(T6 {"Test Progress"=0, "Test Progress Text"=""} ("Progress")) -> ()
        n224 = Index Array(array=w375, index=w374) -> (element=w373:string)
        n225 = call <vilib>:"NT Write String.vi"("String"=w373, "Name"="TestMode/TestName") -> ()  [unwired: 9 in, 1 out]
        n226 = property on="Progress" class="Clust (strict)"("Visible"=TRUE) -> ()  [unwired: 2 in, 2 out]
        n227 = property on="Motor" class="Clust (strict)"("Visible"=w370) -> ()  [unwired: 2 in, 2 out]
        n228 = property on="Test Slider" class="Slide (strict)"("Visible"=w370) -> ()  [unwired: 2 in, 2 out]
        n229 = property on="On/Off" class="Bool (strict)"("Visible"=w370) -> ()  [unwired: 2 in, 2 out]
        n230 = property on="Rev/Fwd" class="Clust (strict)"("Visible"=w370) -> ()  [unwired: 2 in, 2 out]
        n231 = property on="Test Ring" class="Ring (strict)"("Visible"=w370) -> ()  [unwired: 2 in, 2 out]
      }
      event "Select Auto": Mouse Enter {
        # "Populate the combo box with the list of autonomous options"
        n232 = event-data() -> ()  [unwired: 1 in, 1 out]
        n233 = call <vilib>:"NT Read String Array.vi"("Name"="Auto List") -> ("String Array"=w377:string[])  [unwired: 9 in, 1 out]
        n234 = property on="Select Auto" class="CmbBox"("Strings[]"=w377) -> ()  [unwired: 2 in, 2 out]
      }
      event "Select Auto": Value Change {
        # "User modified the Auto Selection. Write to NT variable so robot knows."
        n235 = event-data() -> ("NewVal"=w380:string)  [unwired: 1 in]
        n236 = call <vilib>:"NT Write String.vi"("String"=w380, "Name"="Auto Selector") -> ()  [unwired: 9 in, 1 out]
      }
      event "Command Selection": Value Change {
        # "Get the params and show in table"
        n237 = event-data() -> ("NewVal"=w386:i32)  [unwired: 1 in]
        n238 = property on="Command Selection" class="MCListbox (strict)"() -> ("ItemNames"=w384:string[][])  [unwired: 2 in, 2 out]
        n239 = call <vilib>:"WPI_DashboardUpdate Command Params.vi"("NewVal"=w386, "Commands"=w384, "Param Tbl"=w385) -> ()  [unwired: 8 in, 1 out]
      }
      event "Execute Command": Value Change {
        # "Started one, Unique ID holds\nresponse"
        n240 = event-data() -> ()  [unwired: 1 in, 1 out]
        n241 = property on="Command Selection" class="MCListbox (strict)"() -> ("ItemNames"=w397:string[][])  [unwired: 2 in, 2 out]
        n242 = Index Array(array=w397, index (row)="Command Selection", index (col)=0) -> (element=w395:string)
        n243 = call <vilib>:"Invoke Commands.vi"("Command Params"="Command Params", "Function Name"=w395) -> ("Params"=w391:u8, "Started"=w390:bool)  [unwired: 7 in, 1 out]
        n244 = Array Subset(array="Command Params", length (row)=w391) -> (w392:string[][])  [unwired: 3 in]
        n245 = Select(t="Executing" ("Cmd Status"), s=w390, f="" ("Cmd Status")) -> (s? t:f=→"Cmd Status":string)
      }
      event "Command Selection": Double Click {
        n246 = event-data() -> ("Row"=w405:i32)  [unwired: 1 in]
        n247 = property on="Command Selection" class="MCListbox (strict)"() -> ("ItemNames"=w408:string[][])  [unwired: 2 in, 2 out]
        n248 = local read "Command Params"() -> (w404:string[][])
        n249 = Index Array(array=w408, index (row)=w405, index (col)=0) -> (element=w406:string)
        n250 = call <vilib>:"Invoke Commands.vi"("Command Params"=w404, "Function Name"=w406) -> ("Params"=w403:u8, "Started"=w398:bool)  [unwired: 7 in, 1 out]
        n251 = Array Subset(array=w404, length (row)=w403) -> (w402:string[][])  [unwired: 3 in]
        n252 = Select(t="Executing" ("Cmd Status"), s=w398, f="" ("Cmd Status")) -> (s? t:f=w399:string)
        n253 = local write "Cmd Status"(w399) -> ()
      }
      event "CheckList": Double Click {
        # "Shift clears all"
        # "Update symbols on the listbox"
        n254 = event-data() -> ("PlatMods.Shift"=w410:bool, "Row"=w412:i32)  [unwired: 1 in]
        n255 = case shown="True" w410 {
          tunnel: w412 -> [w416 _]
          tunnel: 1 -> [w415 _]
          frame False {
            n256 = property on="CheckList" class="LstBox (strict)"() -> ("Item Symbols"=w414:i32[])  [unwired: 2 in, 2 out]
            n257 = Replace Array Subset(array=w414, new element=w415, index=w416) -> (w413:i32[])
            n258 = property on="CheckList" class="LstBox (strict)"("Item Symbols"=w413) -> ()  [unwired: 2 in, 2 out]
          }
          frame True {
            w417 = 0 ("Top Row")
            n259 = property on="CheckList" class="LstBox (strict)"() -> ("Number of Rows"=w419:u32)  [unwired: 2 in, 2 out]
            n260 = Initialize Array(0, w419) -> (w418:i32[])
            n261 = property on="CheckList" class="LstBox (strict)"("Top Row"=w417, "Value"=w417, "Item Symbols"=w418) -> ()  [unwired: 2 in, 2 out]
          }
        }
      }
      event "CheckList": Key Down {
        # "Update symbols on the listbox\nLeft and right keys check and uncheck"
        n262 = event-data() -> ("VKey"=w423:T21)  [unwired: 1 in]
        n263 = case shown="\"Left\", \"Right\"" w423 {
          selector: w423 -> [w428 _]
          tunnel: eventvkey."Left" ("VKey") -> [w426 _]
          frame "Left", "Right" {
            n264 = Equal?(x=w426, y=w428) -> (x = y?=w427:bool)
            n265 = Select(t=0, s=w427, f=1) -> (s? t:f=w429:i32)
            n266 = property on="CheckList" class="LstBox (strict)"() -> ("Item Symbols"=w432:i32[])  [unwired: 2 in, 2 out]
            n267 = Replace Array Subset(array=w432, new element=w429, index="CheckList") -> (w431:i32[])
            n268 = property on="CheckList" class="LstBox (strict)"("Item Symbols"=w431) -> ()  [unwired: 2 in, 2 out]
          }
          frame Default {
          }
        }
      }
      event "Motor.Enable": Value Change {
        # "When the test mode otor enable helper is set, update that\ntree row item's value"
        n269 = event-data() -> ("NewVal"=w438:bool)  [unwired: 1 in]
        n270 = Unbundle("Motor") -> ("Value"=w437:dbl)  [unwired: 1 out]
        n271 = Select(t=w437, s=w438, f=0.0) -> (s? t:f=w435:dbl)
        n272 = call <vilib>:"NT Write Number.vi"("Numeric"=w435, "Name"=w434) -> ()  [unwired: 9 in, 1 out]
      }
      event "Test Slider": Value Change {
        # "When the test mode slider helper is set, update that\ntree row item's value"
        n273 = event-data() -> ("NewVal"=w441:dbl)  [unwired: 1 in]
        n274 = call <vilib>:"NT Write Number.vi"("Numeric"=w441, "Name"=w442) -> ()  [unwired: 9 in, 1 out]
      }
      event "On/Off": Value Change {
        # "When the test mode on/off helper value is set, update that\ntree row item's value"
        n275 = event-data() -> ("NewVal"=w446:bool)  [unwired: 1 in]
        n276 = Boolean To (0,1)(Boolean=w446) -> (0, 1=w445:i16)
        n277 = call <vilib>:"NT Write Number.vi"("Numeric"=w445, "Name"=w444) -> ()  [unwired: 9 in, 1 out]
      }
      event "Rev/Fwd": Value Change {
        # "When the test mode helper value for relays is set, update that\ntree row item's value"
        n278 = event-data() -> ("NewVal.Forward"=w454:bool, "NewVal.Reverse"=w453:bool)  [unwired: 1 in]
        n279 = Boolean To (0,1)(Boolean=w454) -> (0, 1=w450:i16)
        n280 = Boolean To (0,1)(Boolean=w453) -> (0, 1=w452:i16)
        n281 = Negate(x=w452) -> (-x=w451:i16)
        n282 = Add(x=w450, y=w451) -> (x+y=w449:i16)
        n283 = call <vilib>:"NT Write Number.vi"("Numeric"=w449, "Name"=w448) -> ()  [unwired: 9 in, 1 out]
      }
      event "Test Ring": Value Change {
        # "When a test mode helper value is selected from the ring,\nset the tree item's variable to the string value"
        n284 = event-data() -> ("NewVal"=w458:u16)  [unwired: 1 in]
        n285 = property on="Test Ring" class="Ring (strict)"() -> ("Strings []"=w459:string[])  [unwired: 2 in, 2 out]
        n286 = Index Array(array=w459, index=w458) -> (element=w457:string)
        n287 = call <vilib>:"NT Write String.vi"("String"=w457, "Name"=w456) -> ()  [unwired: 9 in, 1 out]
      }
      event "Rec Mode": Value Change {
        # "Update globals for recording mode and path to read log from.\nClear when logging and let NetworkTables set path for vision to\nuse."
        n288 = event-data() -> ("NewVal"=w470:enum32{"Stop", "Record", "Playback"})  [unwired: 1 in]
        n289 = global write "WPI_DashboardLogging Global.vi" "Logging Filename"(path "") -> ()
        n290 = global write "WPI_DashboardLogging Global.vi" "Recording"(w470) -> ()
        n291 = case shown="\"Playback\"" w470 {
          tunnel: w469 -> [_ w472 w481]
          tunnel: [_ _ w480] -> w467
          tunnel: [_ _ w479] -> _
          tunnel: w465 -> [_ _ w477]
          tunnel: cluster{i32, i32} {-250, 170} -> [_ _ w476]
          tunnel: [_ _ T22 {"Image Size"=TRUE, "Image Type"=TRUE, "Pixel Value"=TRUE, "ROI Information"=TRUE, "Zoom Factor"=FALSE} ("Image Information Shown:All Elements")] -> w460
          tunnel: [_ _ TRUE ("Zoom Factor")] -> w461
          tunnel: w463 -> [_ _ w473]
          frame Default {
          }
          frame "Stop", "Record" {
            # "Place Window too"
            n292 = invoke class="VI" method="FP.Close"(reference=w472) -> (reference out=w471:refnum<vi>)  [unwired: 2 in, 2 out]
            n293 = invoke class="VI" method="Abort VI"(reference=w471) -> ()  [unwired: 2 in, 3 out]
          }
          frame "Playback" {
            n294 = call "Open Playback Panel.vi"("Offset"=w476, "DB VI Ref"=w477, "Playback in"=w481) -> ("Playback out"=w478:refnum<vi>)  [unwired: 8 in]
            n295 = register-events(w478, w473) -> (reference out=w480:refnum<event-registration>, error out=w479:errorcluster)  [unwired: 2 in]
          }
        }
        n296 = property on="Camera Image Right" class="ImageControl"("Image Information Shown"=w460, "Image Information Visible"=w461) -> ()  [unwired: 2 in, 2 out]
        n297 = property on="Camera Image" class="ImageControl"("Image Information Shown"=w460, "Image Information Visible"=w461) -> ()  [unwired: 2 in, 2 out]
        n298 = call <vilib>:"WPI_DashboardNT Log FieldName Cache.vi"("Operation"=enum16{"Lookup/Add", "Index", "Clear"}."Clear") -> ()  [unwired: 8 in, 3 out]
      }
      event Panel Close {
        w483 = enum32{"Stop", "Record", "Playback"}."Stop" ("Rec Mode")
        # "Playback window has been closed, abort"
        n299 = event-data() -> ()  [unwired: 1 in, 4 out]
        n300 = local write "Rec Mode"(w483) -> ()
        n301 = global write "WPI_DashboardLogging Global.vi" "Recording"(w483) -> ()
      }
      event Panel Close {
        # "Abort playback window and ourself"
        n302 = event-data() -> ()  [unwired: 1 in, 4 out]
        n303 = invoke class="VI" method="FP.Close"(reference=w487) -> (reference out=w486:refnum<vi>)  [unwired: 2 in, 2 out]
        n304 = invoke class="VI" method="Abort VI"(reference=w486) -> (error out=w485:errorcluster)  [unwired: 2 in, 2 out]
        n305 = invoke class="VI" method="Abort VI"(error in=w485) -> ()  [unwired: 2 in, 3 out]
      }
      event User Event {
        n306 = event-data() -> ("IDs"=w494:cluster{"RPC field ID":u16, "Unique ID":u16}, "String"=w493:string)  [unwired: 1 in]
        n307 = Bundle("IDs"=w494, "String"=w493) -> (w492:T9)  [unwired: 1 in]
        n308 = call <vilib>:"Retrieve RPC Response.vi"("RPC Response"=w492) -> ("Output"=w490:string[][])  [unwired: 10 in]
        n309 = Build Array (concatenate)(w488, w490) -> (w489:string[][])
        n310 = local write "Command Params"(w489) -> ()
        n311 = local write "Cmd Status"("" ("Cmd Status")) -> ()
      }
      event "Tree": Double Click {
        n312 = event-data() -> ("PlatMods"=w500:T25, "Tag"=w497:string)  [unwired: 1 in]
        n313 = Unbundle(w500) -> ("Shift"=w499:bool)  [unwired: 4 out]
        n314 = String Subset(string=w497, length (rest)=1 ("length (rest)")) -> (substring=w496:string)  [unwired: 1 in]
        n315 = Not(x=w499) -> (.not. x?=w498:bool)
        n316 = case shown="\"/\"" w496 {
          tunnel: w497 -> [_ w503]
          tunnel: w498 -> [_ w502]
          frame Default {
          }
          frame "/" {
            n317 = call <vilib>:"NT Update Persistence.vi"("Persistence"=w502, "Name"=w503) -> ()  [unwired: 9 in, 1 out]
          }
        }
      }
    }
  }
  n318 = while {
    tunnel: w65 -> [w505]
    i -> [w508]
    stop <- FALSE stop-if-true
    n319 = Wait (ms)(milliseconds to wait=u32 100) -> ()  [unwired: 1 out]
    n320 = case shown="\"Playback\"" "Rec Mode" {
      tunnel: w508 -> [_ _ w523]
      tunnel: [u32 2829099 ("Base Color") u32 11141120 ("Target Color") w512] -> w504
      frame "Stop", Default {
        # "Reset the color, extra updates don't cost much"
      }
      frame "Record" {
      }
      frame "Playback" {
        # "Playback"
        n321 = Quotient & Remainder(x=w523, y=u32 50 ("milliseconds to wait")) -> (x-y*floor(x/y)=w519:u32)  [unwired: 1 out]
        n322 = Divide(x=w519, y=u32 50 ("milliseconds to wait")) -> (x/y=w516:dbl)
        n323 = Multiply(x=6.283185307179586, y=w516) -> (x*y=w521:dbl)
        n324 = Sine(x=w521) -> (sin(x)=w520:dbl)
        n325 = Absolute Value(x=w520) -> (abs(x)=w513:dbl)
        n326 = call "Interpolate RGB Color.vi"("Proportion"=w513, "Target Color"=u32 30976, "Base Color"=u32 2829099) -> ("Result Color"=w512:u32)  [unwired: 8 in]
      }
    }
    n327 = property class="Pane"(reference=w505, "PaneColor"=w504) -> ()  [unwired: 1 in, 2 out]
  }
  n328 = local write "Dashboard Tab"(T2."Drive" ("Dashboard Tab")) -> ()
  n329 = property on="On/Off" class="Bool (strict)"("Visible"=w36) -> ()  [unwired: 2 in, 2 out]
  n330 = property on="Motor" class="Clust (strict)"("Visible"=w36) -> ()  [unwired: 2 in, 2 out]
  n331 = property on="Progress" class="Clust (strict)"("Visible"=w36) -> ()  [unwired: 2 in, 2 out]
  n332 = property on="Test Ring" class="Ring (strict)"("Visible"=w36) -> ()  [unwired: 2 in, 2 out]
  n333 = property on="Rev/Fwd" class="Clust (strict)"("Visible"=w36) -> ()  [unwired: 2 in, 2 out]
  n334 = while {
    tunnel: u16 1741 ("timeout ms (25000)") -> [w525]
    stop <- FALSE stop-if-true
    n335 = TCP Create Listener(10:w525) -> (0:w524:errorcluster, 3:w526:refnum<k5>)  [unwired: 4 in, 1 out]
    n336 = case shown="No Error" w524 {
      selector: w524 -> [w528 _]
      tunnel: w526 -> [w529 _]
      frame No Error {
        n337 = while {
          tunnel: w529 -> [w532]
          tunnel: w528 -> [w531]
          stop <- FALSE stop-if-true
          n338 = TCP Wait On Listener(8:w531, 11:w532) -> (0:w533:errorcluster, 4:w534:refnum<k5>)  [unwired: 2 in, 3 out]
          n339 = local write "TCP"(w534) -> ()
          n340 = case shown="No Error" w533 {
            frame No Error {
            }
            frame Error {
              n341 = Wait (ms)(milliseconds to wait=u32 1000) -> ()  [unwired: 1 out]
            }
          }
        }
      }
      frame Error {
        n342 = Wait (ms)(milliseconds to wait=u32 1000) -> ()  [unwired: 1 out]
      }
    }
  }
  n343 = local write "Command Selection"(u16 0 ("milliseconds to wait")) -> ()
  n344 = local write "Command Params"(string[][] [] ("Command Params")) -> ()
  n345 = global write "WPI_DashboardLogging Global.vi" "Recording"(w59) -> ()
  n346 = local write "Rec Mode"(w59) -> ()
  n347 = call <vilib>:"NT Write String.vi"("String"="Select Auto", "Name"="Auto Selector") -> ()  [unwired: 9 in, 1 out]
